vi "stoperaseAO_tt.vi"   [LabVIEW 2013]
types:
  T1 = typedef "LVRectTypeDef.ctl" = cluster{"Left":i16, "Top":i16, "Right":i16, "Bottom":i16}
  T2 = cluster{"Xpixels":i32, "Vxminref":dbl, "Vxmaxref":dbl, "P":dbl, "Ypixels":i32, "Vyminref":dbl, "Vymaxref":dbl, "srate":sgl, "sAOxy":i32, "timeout":dbl, "type":string, "date":string, "time":string, "Colormap":u16, "Drawing Mode":u16, "Scanning Mode":u16, "square pixels":bool, "square matrix":bool, "Xpixels Img":i32, "Vx-min Img":dbl, "VX-max Img":dbl, "Ypixels Img":i32, "Vy-min Img":dbl, "Vy-max Img ":dbl, "Angle Img":dbl, "autoshutter":bool, "finite":bool, "cont":bool, "wavdet":bool, "measpoints":i32, "avpp":i32, "bufferAO":i32, "bufferAI":i32, "starttick":u32, "waveform":path, "Vx-ref":dbl, "Vy-ref":dbl, "refreshrate":dbl, "refreshbuffer":i32, "tt_cycles":i32, "motorref":refnum<k7>, "mirrorswitch":refnum<k7>, "sample mode":i32, "maxbufferAI":i32, "sampletreshold":dbl, "srateAODO":sgl, "bin":sgl, "Pel":sgl, "Angle draw":dbl, "srate Img":sgl, "ROIimg_plotbounds":T1, "auto OD":bool, "ODfilt":u16, "reset AO_DO":bool, "aAI":i32[], "aCI":i32[], "aAO":i32[], "aDO":i32[]}
  T3 = cluster{"Min Voltage sq (mV)":dbl, "Max voltage sq (mV)":dbl, "Duty cycle sq(%)":dbl, "Voltage freq. sq(Hz)":dbl, "# cycles sq":u32, "meastype":enum16{"sealtest hekcells", "sealtest neurons", "Manual", "from file"}, "sample rate":dbl, "amp":dbl, "sample mode":i32, "refreshbuffer":i32, "timeout":sgl, "Min Voltage tri (mV)":dbl, "Max voltage tri (mV)":dbl, "Voltage freq. tri(Hz)":dbl, "# cycles tri":u32, "Voltage step ":bool, "Voltage triangle":bool, "file":bool, "refreshrate":dbl, "sAOXY":dbl, "avpp":i32, "Pel":dbl, "bin":dbl, "lAO":i32[], "lDO":i32[]}
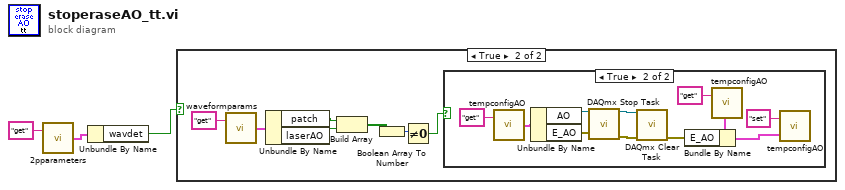
[diagram p0: block diagram]
diagram:
  n1 = call "2pparameters.vi"("command"="get") -> ("params out"=w3:T2)  [unwired: 1 in]
  n2 = Unbundle By Name(w3) -> ("wavdet"=w1:bool)
  n3 = case shown="True" w1 {
    frame False {
    }
    frame True {
      n4 = call "waveformparams.vi"("command"="get") -> ("Params out"=w6:T3)  [unwired: 1 in]
      n5 = Unbundle By Name(w6) -> ("patch"=w7:bool, "laserAO"=w8:bool)
      n6 = Build Array(w7, w8) -> (w9:bool[])
      n7 = Boolean Array To Number(Boolean array=w9) -> (number=w10:u32)
      n8 = Not Equal To 0?(x=w10) -> (x != 0?=w4:bool)
      n9 = case shown="True" w4 {
        frame False {
        }
        frame True {
          n10 = call "tempconfigAO.vi"("command"="get") -> ("Temp Config out"=w18:cluster{"AO":refnum<k21>, "E_AO":errorcluster})  [unwired: 1 in]
          n11 = Unbundle By Name(w18) -> ("AO"=w17:refnum<k21>, "E_AO"=w16:errorcluster)
          n12 = call <vilib>:"DAQmx Stop Task.vi"("task/channels in"=w17, "error in"=w16) -> ("task out"=w20:refnum<k21>, "error out"=w21:errorcluster)  [unwired: 12 in]
          n13 = call <vilib>:"DAQmx Clear Task.vi"("task in"=w20, "error in"=w21) -> ("error out"=w12:errorcluster)  [unwired: 13 in]
          n14 = call "tempconfigAO.vi"("command"="get") -> ("Temp Config out"=w13:cluster{"AO":refnum<k21>, "E_AO":errorcluster})  [unwired: 1 in]
          n15 = Bundle By Name(cluster=w13, "E_AO"=w12) -> (w11:cluster{"AO":refnum<k21>, "E_AO":errorcluster})
          n16 = call "tempconfigAO.vi"("Temp Config in"=w11, "command"="set") -> ()  [unwired: 1 out]
        }
      }
    }
  }
